vi "Generate Excel Report.vi"() -> ()   [LabVIEW 2018]
doc: "This example shows how to generate a report from a template. The template contains a preformatted table and a preformatted graph which are updated with Append Table to Report.vi and Excel Update Graph.vi."
uses:
  <vilib>/Utility/NIReport.llb/Append Report Text (str wrap).vi
  <vilib>/Utility/NIReport.llb/Append Text Table to Report (wrap).vi
  <vilib>/Utility/NIReport.llb/NI_report.lvclass
  <vilib>/Utility/NIReport.llb/Excel/NI_Excel.lvclass
panel:
  in  "Additional Report Values":T1(array[cluster])
  in  "template (empty)":path
  in  "Safe to Path":path
  in  "Test operator":string="Operator's name"
  in  "Pressure":string="100"
  in  "Humidity":string="70"
  in  "Temperature":string="20"
  in  "Data":string[][](table)=[["100", "41.7", "38.5"], ["125", "41.7", "35.2"], ["160", "41.5", "37.5"], ["200", "42.3", "42.5"], ["250", "46.9", "46.8"], ["315", "51.9", "52.6"], ["400", "52.3", "46.7"], ["500  ", "46.5", "41.6"], ["630", "42.3", "35.9"], ["800", "41.1", "32.6"]]
  # "This example shows how to generate a report from a template using either the Excel Report Generation VIs or the MS Office Report Express VI. The template contains several named cells which are used to place data in the appropriate positions in the template."
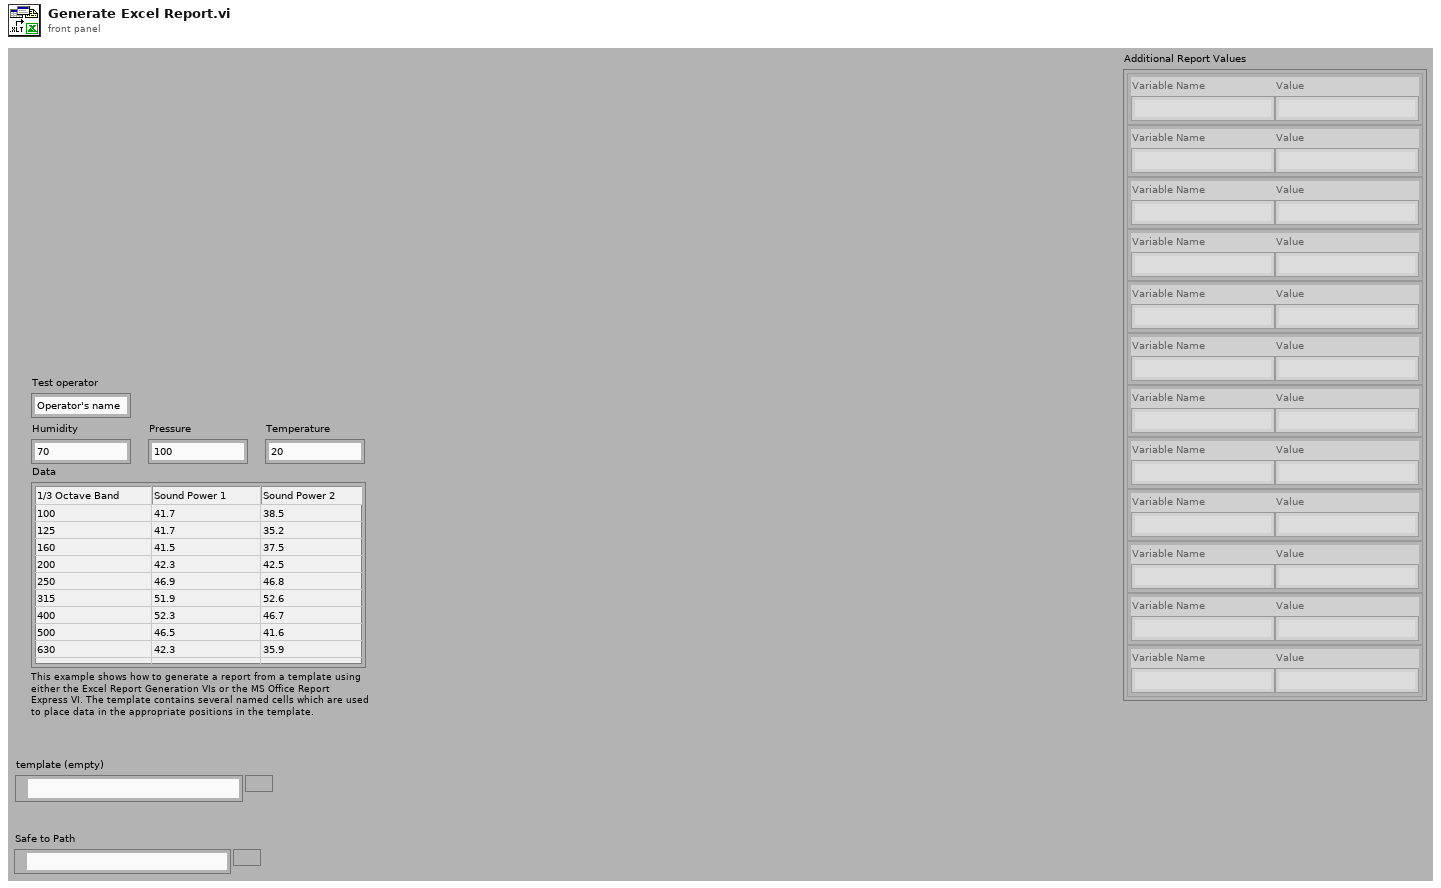
[diagram p1: front panel]
types:
  T1 = cluster{"Variable Name":string, "Value":string}[]
  T2 = cluster{"position (Excel)":cluster{"row":i32, "column":i32}, "name (Excel)":string, "bookmark (Word)":string}
  T3 = enum16{"Standard Report", "HTML", "Word", "Excel"}
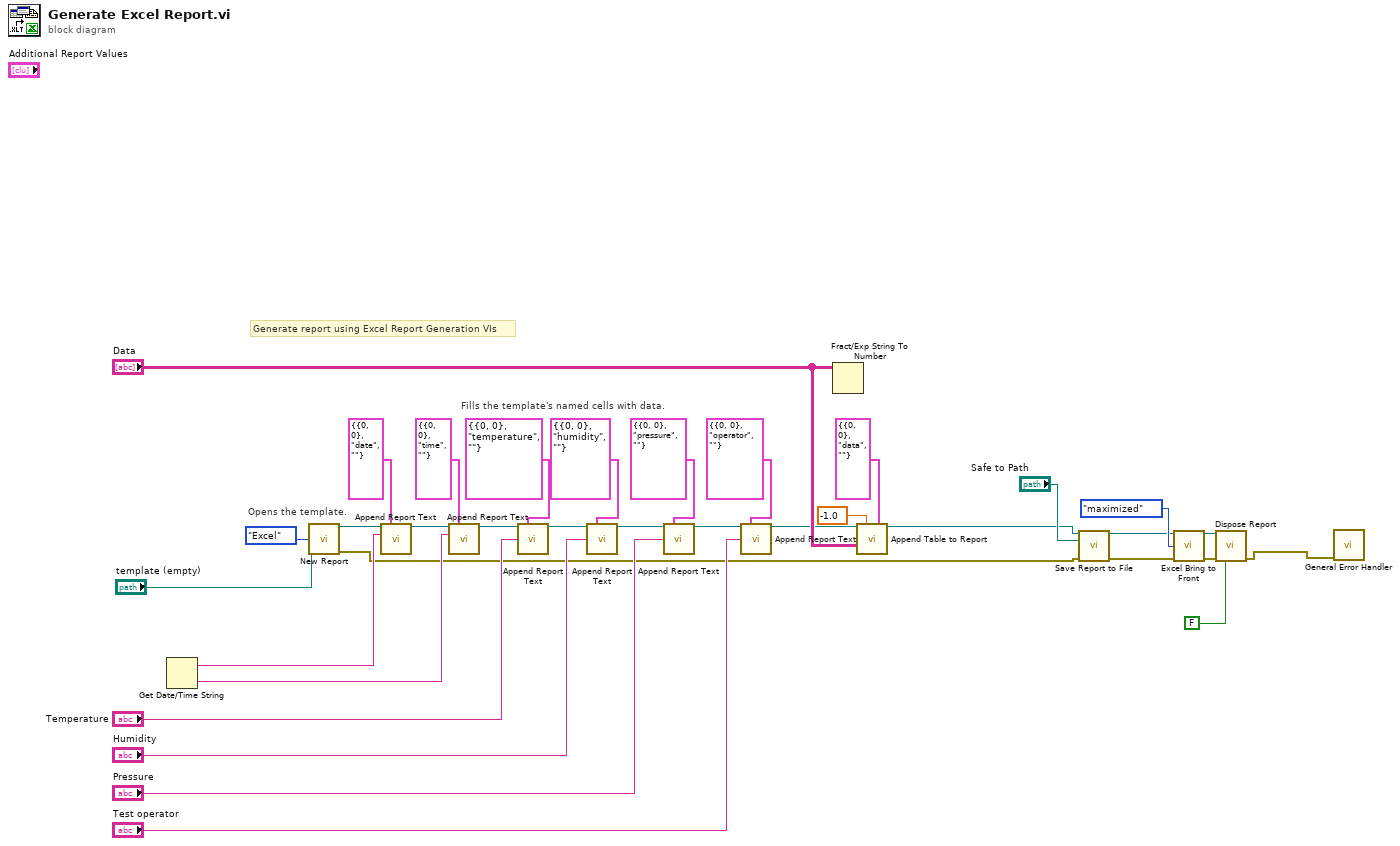
[diagram p0: block diagram]
diagram:
  # "Generate report using Excel Report Generation VIs"
  # "Fills the template's named cells with data."
  # "Opens the template."
  n1 = Get Date/Time String() -> (date string=w34:string, time string=w33:string)  [unwired: 3 in]
  n2 = call <vilib>:"New Report.vi"("report type"=T3."Excel", "template (empty)"="template (empty)") -> ("report out"=w25:refnum<class "NI_report.lvclass">, "error out"=w4:errorcluster)  [unwired: 12 in]
  n3 = call-poly <vilib>:"Append Report Text.vi"("report in"=w25, "MS Office parameters"=T2 {"position (Excel)"={"row"=0, "column"=0}, "name (Excel)"="date", "bookmark (Word)"=""}, "text"=w34) -> ("report out"=w24:refnum<class "NI_report.lvclass">)  [unwired: 9 in, 3 out]
  n4 = call-poly <vilib>:"Append Report Text.vi"("report in"=w24, "MS Office parameters"=T2 {"position (Excel)"={"row"=0, "column"=0}, "name (Excel)"="time", "bookmark (Word)"=""}, "text"=w33) -> ("report out"=w23:refnum<class "NI_report.lvclass">)  [unwired: 9 in, 3 out]
  n5 = call-poly <vilib>:"Append Report Text.vi"("report in"=w23, "MS Office parameters"=T2 {"position (Excel)"={"row"=0, "column"=0}, "name (Excel)"="temperature", "bookmark (Word)"=""}, "text"="Temperature") -> ("report out"=w22:refnum<class "NI_report.lvclass">)  [unwired: 9 in, 3 out]
  n6 = call-poly <vilib>:"Append Report Text.vi"("report in"=w22, "MS Office parameters"=T2 {"position (Excel)"={"row"=0, "column"=0}, "name (Excel)"="humidity", "bookmark (Word)"=""}, "text"="Humidity") -> ("report out"=w21:refnum<class "NI_report.lvclass">)  [unwired: 9 in, 3 out]
  n7 = call-poly <vilib>:"Append Report Text.vi"("report in"=w21, "MS Office parameters"=T2 {"position (Excel)"={"row"=0, "column"=0}, "name (Excel)"="pressure", "bookmark (Word)"=""}, "text"="Pressure") -> ("report out"=w20:refnum<class "NI_report.lvclass">)  [unwired: 9 in, 3 out]
  n8 = call-poly <vilib>:"Append Report Text.vi"("report in"=w20, "MS Office parameters"=T2 {"position (Excel)"={"row"=0, "column"=0}, "name (Excel)"="operator", "bookmark (Word)"=""}, "text"="Test operator") -> ("report out"=w19:refnum<class "NI_report.lvclass">)  [unwired: 9 in, 3 out]
  n9 = Fract/Exp String To Number(string="Data") -> ()  [unwired: 3 in, 2 out]
  n10 = call-poly <vilib>:"Append Table to Report.vi"("report in"=w19, "column width (1)"=-1.0, "MS Office parameters"=T2 {"position (Excel)"={"row"=0, "column"=0}, "name (Excel)"="data", "bookmark (Word)"=""}, "text data"="Data") -> ("report out"=w3:refnum<class "NI_report.lvclass">)  [unwired: 8 in, 3 out]
  n11 = call-dynamic "Save Report to File.vi"("report in"=w3, "report file path"="Safe to Path", "error in (no error)"=w4) -> ("report out"=w1:refnum<class "NI_report.lvclass">, "error out"=w2:errorcluster)  [unwired: 11 in]
  n12 = call <vilib>:"Excel Bring to Front.vi"("report in"=w1, "window state (maximized)"=enum16{"maximized", "minimized", "normal"}."maximized", "error in (no error)"=w2) -> ("report out"=w8:refnum<class "NI_report.lvclass">, "error out"=w7:errorcluster)  [unwired: 11 in]
  n13 = call-dynamic "Dispose Report.vi"("report in"=w8, "error in (no error)"=w7, "close report? (T)"=FALSE ("Close Report? (T)")) -> ("error out"=w27:errorcluster)  [unwired: 12 in]
  n14 = call <vilib>:"General Error Handler.vi"("error in (no error)"=w27) -> ()  [unwired: 10 in, 5 out]
